vi "jMsg_SnakeProcessor_StopGame (create).vi"(8 "error in (no error)":errorcluster) -> (0 "error out":errorcluster, 3 "jMsg_SnakeProcessor_StopGame":refnum<class "jMsg_SnakeProcessor_StopGame.lvclass">)   [LabVIEW 2019, in "jMsg_SnakeProcessor_StopGame.lvclass"]
doc: "This VI is used to create the jMsg\n\n\nJSMA Message Wizard 0.2.0.5\nRob Humfeld - Jet Engineering\nCopyright (c) 2020, Jet Engineering"
uses:
  jMsg_SnakeProcessor_StopGame.lvclass
  C:/Program Files/National Instruments/LabVIEW 2019/user.lib/Jet Engineering/JSMA/Libraries/jMsg Class/jMsg.lvclass
  <userlib>/Jet Engineering/JSMA/Libraries/jMsg Class/jMsg.lvclass/jMsg.ctl
  <userlib>/Jet Engineering/JSMA/Libraries/Shared/JSMA_GetClassName.vi
  <vilib>/Utility/LVClass/Get LV Class Path.vi
  <userlib>/Jet Engineering/JSMA/Libraries/jMsg Class/jMsg.lvclass
panel:
  in  "jMsg_SnakeProcessor_StopGame":refnum<class "jMsg_SnakeProcessor_StopGame.lvclass">
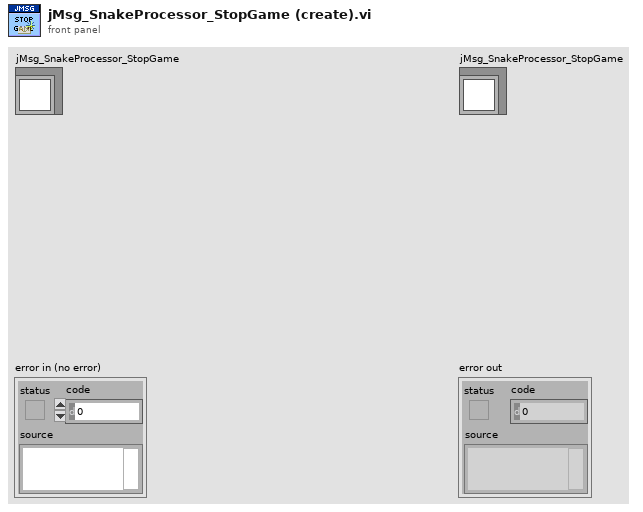
[diagram p1: front panel]
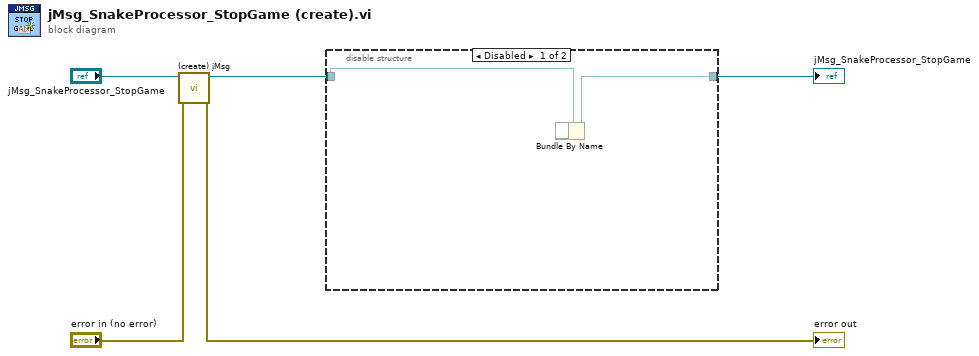
[diagram p0: block diagram]
diagram:
  n1 = call <userlib>:"(create) jMsg.vi"("error in (no error)"="error in (no error)", "jMsg in"="jMsg_SnakeProcessor_StopGame") -> ("error out"=→"error out":errorcluster, "jMsg out"=w1:refnum<class "jMsg_SnakeProcessor_StopGame.lvclass">)  [unwired: 8 in]
  n2 = disable-structure shown="Disabled" {
    disable-tunnel: w1 -> [w7 w8]
    disable-tunnel: [w6 w8] -> w5
    frame Disabled {
      n3 = Bundle By Name(cluster=w7) -> (w6:refnum<class "jMsg_SnakeProcessor_StopGame.lvclass">)  [unwired: 1 in]
    }
    frame Enabled {
    }
  }
  "jMsg_SnakeProcessor_StopGame" <- w5
